vi "LONG_ASCII (SubVI).vi"(1 "String in":string) -> (0 "String out":string)   [LabVIEW 8.6]
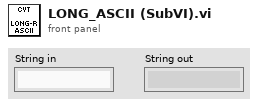
[diagram p1: front panel]
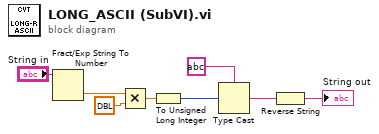
[diagram p0: block diagram]
diagram:
  n1 = Fract/Exp String To Number(string="String in") -> (number=w4:dbl)  [unwired: 3 in, 1 out]
  n2 = Multiply(x=w4, y=dbl ?) -> (x*y=w6:dbl)
  n3 = To Unsigned Long Integer(number=w6) -> (unsigned 32bit integer=w1:u32)
  n4 = Type Cast(type=string ?, x=w1) -> (*(type *) &x=w7:string)
  n5 = Reverse String(1:w7) -> (0:→"String out":string)
